vi "DashboardGetvi.vi"(8 "Joystick 2":T1, 9 "Joystick 1":T1) -> ()   [LabVIEW 2018]
uses:
  <vilib>/Rock Robotics/WPI/Joystick/WPI_JoystickDevRef.ctl
  <vilib>/Rock Robotics/WPI/Joystick/WPI_JoystickDeviceEnum.ctl
  <vilib>/Rock Robotics/Network Tables/NT Read Boolean.vi
  <vilib>/Rock Robotics/Network Tables/NT Read Number.vi
  Inputs_DriverStation.vi
  RobotStates.vi
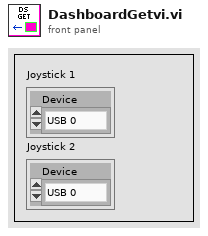
[diagram p1: front panel]
types:
  T1 = typedef "WPI_JoystickDevRef.ctl" = cluster{"Device":T2}
  T2 = typedef "WPI_JoystickDeviceEnum.ctl" = enum16{"USB 0", "USB 1", "USB 2", "USB 3", "USB 4", "USB 5"}
  T3 = cluster{bool, bool, bool, bool, bool, bool, bool, bool, bool, bool, bool, bool, bool, bool}
  T4 = cluster{"Boolean":bool, "Boolean":bool, "Boolean":bool, "Boolean":bool, "Boolean":bool, "Boolean":bool, "Boolean":bool, "Boolean":bool, "Boolean":bool, "Boolean":bool, "Boolean":bool, "Boolean":bool, "Boolean":bool, "Boolean":bool}
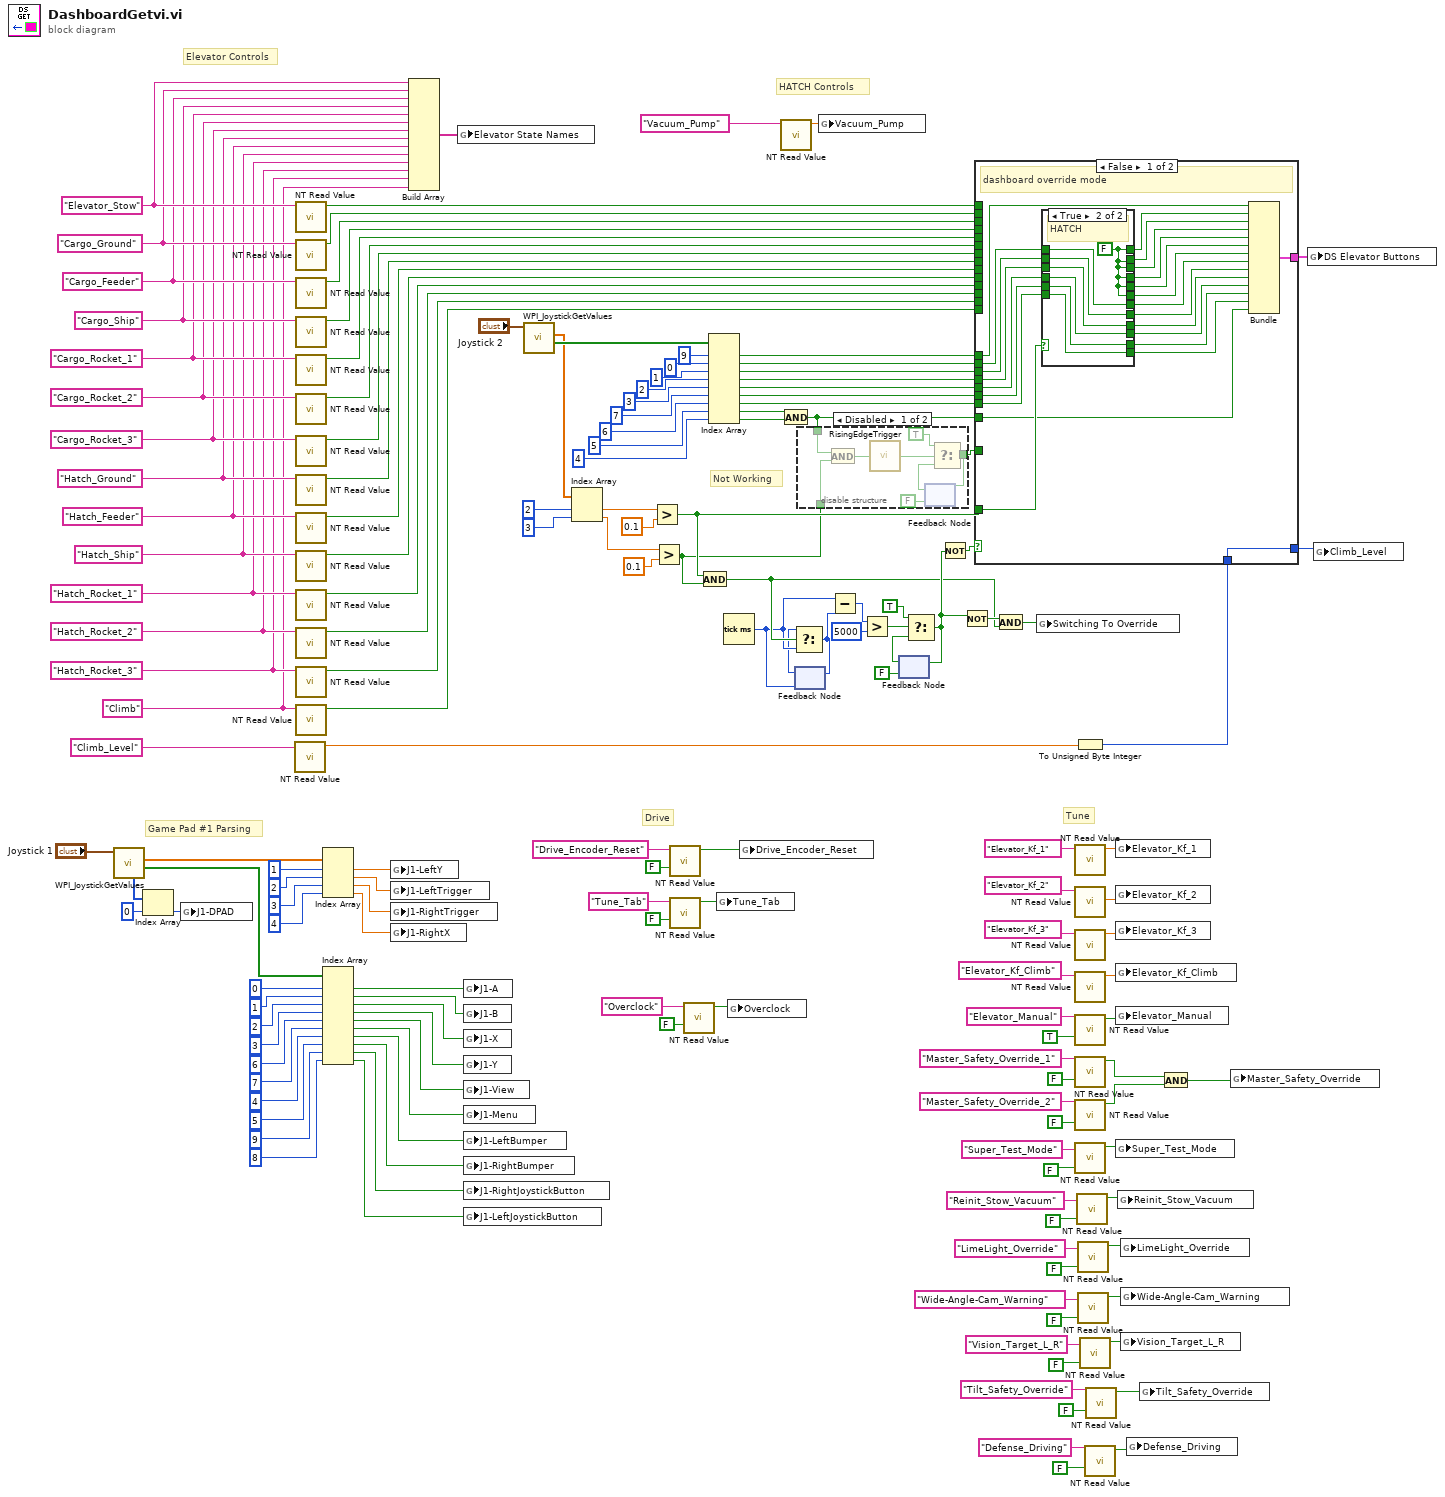
[diagram p0: block diagram]
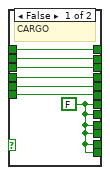
[diagram p3: hidden frame]
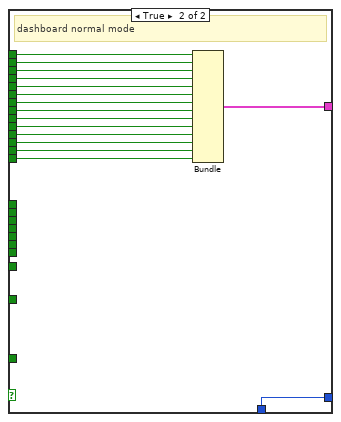
[diagram p4: hidden frame]
diagram:
  w92 = "Climb" ("refnum name")
  w100 = "Hatch_Rocket_3" ("refnum name")
  w101 = "Hatch_Rocket_2" ("refnum name")
  w102 = "Hatch_Rocket_1" ("refnum name")
  w103 = "Hatch_Ship" ("refnum name")
  w104 = "Hatch_Feeder" ("refnum name")
  w105 = "Hatch_Ground" ("refnum name")
  w149 = "Cargo_Rocket_3" ("refnum name")
  w150 = "Cargo_Rocket_2" ("refnum name")
  w151 = "Cargo_Rocket_1" ("refnum name")
  w152 = "Cargo_Ship" ("refnum name")
  w158 = "Cargo_Feeder" ("refnum name")
  w159 = "Cargo_Ground" ("refnum name")
  w160 = "Elevator_Stow" ("refnum name")
  # "Not Working"
  # "Tune"
  # "Drive"
  # "HATCH Controls"
  # "Game Pad #1 Parsing"
  # "Elevator Controls"
  n1 = call <vilib>:"WPI_JoystickGetValues.vi"("JoystickDevRef"="Joystick 1") -> ("Buttons"=w140:bool[], "Axes"=w139:dbl[], "POVs"=w136:i16[])  [unwired: 6 in, 2 out]
  n2 = Index Array(array=w136, index=0) -> (element=w133:i16)
  n3 = global write "Inputs_DriverStation.vi" "J1-DPAD"(w133) -> ()
  n4 = call-poly <vilib>:"NT Read Value.vi"("Name"="Climb_Level" ("refnum name")) -> ("Numeric"=w9:dbl)  [unwired: 9 in, 1 out]
  n5 = call-poly <vilib>:"NT Read Value.vi"("Name"=w160) -> ("Boolean"=w163:bool)  [unwired: 9 in, 1 out]
  n6 = call-poly <vilib>:"NT Read Value.vi"("Name"=w159) -> ("Boolean"=w162:bool)  [unwired: 9 in, 1 out]
  n7 = call-poly <vilib>:"NT Read Value.vi"("Name"=w158) -> ("Boolean"=w161:bool)  [unwired: 9 in, 1 out]
  n8 = call-poly <vilib>:"NT Read Value.vi"("Name"=w152) -> ("Boolean"=w156:bool)  [unwired: 9 in, 1 out]
  n9 = call-poly <vilib>:"NT Read Value.vi"("Name"=w151) -> ("Boolean"=w155:bool)  [unwired: 9 in, 1 out]
  n10 = call-poly <vilib>:"NT Read Value.vi"("Name"=w150) -> ("Boolean"=w154:bool)  [unwired: 9 in, 1 out]
  n11 = call-poly <vilib>:"NT Read Value.vi"("Name"=w149) -> ("Boolean"=w153:bool)  [unwired: 9 in, 1 out]
  n12 = call-poly <vilib>:"NT Read Value.vi"("Name"=w105) -> ("Boolean"=w112:bool)  [unwired: 9 in, 1 out]
  n13 = call-poly <vilib>:"NT Read Value.vi"("Name"=w104) -> ("Boolean"=w111:bool)  [unwired: 9 in, 1 out]
  n14 = call-poly <vilib>:"NT Read Value.vi"("Name"=w103) -> ("Boolean"=w110:bool)  [unwired: 9 in, 1 out]
  n15 = call-poly <vilib>:"NT Read Value.vi"("Name"=w102) -> ("Boolean"=w109:bool)  [unwired: 9 in, 1 out]
  n16 = call-poly <vilib>:"NT Read Value.vi"("Name"=w101) -> ("Boolean"=w108:bool)  [unwired: 9 in, 1 out]
  n17 = call-poly <vilib>:"NT Read Value.vi"("Name"=w100) -> ("Boolean"=w107:bool)  [unwired: 9 in, 1 out]
  n18 = call-poly <vilib>:"NT Read Value.vi"("Name"=w92) -> ("Boolean"=w91:bool)  [unwired: 9 in, 1 out]
  n19 = Index Array(array=w139, index #1=1 ("index"), index #2=2 ("index"), index #3=3 ("index"), index #4=4 ("index")) -> (element #1=w126:dbl, element #2=w127:dbl, element #3=w128:dbl, element #4=w125:dbl)
  n20 = Index Array(array=w140, index #1=0 ("index"), index #2=1 ("index"), index #3=2 ("index"), index #4=3 ("index"), index #5=6 ("index"), index #6=7 ("index"), index #7=4 ("index"), index #8=5 ("index"), index #9=9 ("index"), index #10=8 ("index")) -> (element #1=w132:bool, element #2=w131:bool, element #3=w130:bool, element #4=w129:bool, element #5=w89:bool, element #6=w85:bool, element #7=w82:bool, element #8=w81:bool, element #9=w79:bool, element #10=w74:bool)
  n21 = global write "Inputs_DriverStation.vi" "J1-LeftY"(w126) -> ()
  n22 = global write "Inputs_DriverStation.vi" "J1-LeftTrigger"(w127) -> ()
  n23 = global write "Inputs_DriverStation.vi" "J1-RightTrigger"(w128) -> ()
  n24 = global write "Inputs_DriverStation.vi" "J1-RightX"(w125) -> ()
  n25 = Build Array(w160, w159, w158, w152, w151, w150, w149, w105, w104, w103, w102, w101, w100, w92) -> (w157:string[])
  n26 = global write "RobotStates.vi" "Elevator State Names"(w157) -> ()
  n27 = global write "Inputs_DriverStation.vi" "J1-A"(w132) -> ()
  n28 = global write "Inputs_DriverStation.vi" "J1-B"(w131) -> ()
  n29 = global write "Inputs_DriverStation.vi" "J1-X"(w130) -> ()
  n30 = global write "Inputs_DriverStation.vi" "J1-Y"(w129) -> ()
  n31 = global write "Inputs_DriverStation.vi" "J1-View"(w89) -> ()
  n32 = global write "Inputs_DriverStation.vi" "J1-Menu"(w85) -> ()
  n33 = global write "Inputs_DriverStation.vi" "J1-LeftBumper"(w82) -> ()
  n34 = global write "Inputs_DriverStation.vi" "J1-RightBumper"(w81) -> ()
  n35 = global write "Inputs_DriverStation.vi" "J1-RightJoystickButton"(w79) -> ()
  n36 = global write "Inputs_DriverStation.vi" "J1-LeftJoystickButton"(w74) -> ()
  n37 = call <vilib>:"WPI_JoystickGetValues.vi"("JoystickDevRef"="Joystick 2") -> ("Buttons"=w69:bool[], "Axes"=w53:dbl[])  [unwired: 6 in, 3 out]
  n38 = Index Array(array=w53, index #1=2 ("index"), index #2=3 ("index")) -> (element #1=w52:dbl, element #2=w48:dbl)
  n39 = Greater?(x=w52, y=0.1) -> (0:w47:bool)
  n40 = Greater?(x=w48, y=0.1) -> (0:w35:bool)
  n41 = call-poly <vilib>:"NT Read Value.vi"("Default Value"=FALSE, "Name"="Drive_Encoder_Reset" ("refnum name")) -> ("Boolean"=w113:bool)  [unwired: 8 in, 1 out]
  n42 = call-poly <vilib>:"NT Read Value.vi"("Default Value"=FALSE, "Name"="Tune_Tab" ("refnum name")) -> ("Boolean"=w76:bool)  [unwired: 8 in, 1 out]
  n43 = call-poly <vilib>:"NT Read Value.vi"("Default Value"=FALSE, "Name"="Overclock" ("refnum name")) -> ("Boolean"=w23:bool)  [unwired: 8 in, 1 out]
  n44 = And(x=w47, y=w35) -> (x .and. y?=w29:bool)
  n45 = Index Array(array=w69, index #1=9 ("index"), index #2=0 ("index"), index #3=1 ("index"), index #4=2 ("index"), index #5=3 ("index"), index #6=7 ("index"), index #7=6 ("index"), index #8=5 ("index"), index #9=4 ("index")) -> (element #1=w67:bool, element #2=w65:bool, element #3=w63:bool, element #4=w61:bool, element #5=w59:bool, element #6=w57:bool, element #7=w55:bool, element #8=w38:bool, element #9=w37:bool)
  n46 = global write "Inputs_DriverStation.vi" "Tune_Tab"(w76) -> ()
  n47 = Tick Count (ms)() -> (millisecond timer value=w27:u32)
  n48 = global write "Inputs_DriverStation.vi" "Overclock"(w23) -> ()
  n49 = global write "Inputs_DriverStation.vi" "Drive_Encoder_Reset"(w113) -> ()
  n50 = call-poly <vilib>:"NT Read Value.vi"("Name"="Vacuum_Pump" ("refnum name")) -> ("Numeric"=w116:dbl)  [unwired: 9 in, 1 out]
  n51 = And(x=w38, y=w37) -> (x .and. y?=w36:bool)
  n52 = feedback #1(w27) -> (w26:u32)
  n53 = Select(t=w26, s=w29, f=w27) -> (s? t:f=w33:u32)
  n54 = feedback-in #1(w33) -> ()
  n55 = disable-structure shown="Disabled" {
    disable-tunnel: w36 -> [w171 _]
    disable-tunnel: w35 -> [w170 _]
    disable-tunnel: [w164 _] -> w34
    frame Disabled {
      n56 = And(x=w171, y=w170) -> (x .and. y?=w169:bool)
      n57 = call "RisingEdgeTrigger.vi"("Raw Signal"=w169) -> ("Trigger"=w165:bool)
      n58 = feedback #2(FALSE) -> (w167:bool)
      n59 = Select(t=TRUE, s=w165, f=w167) -> (s? t:f=w164:bool)
      n60 = feedback-in #2(w164) -> ()
    }
    frame Enabled {
    }
  }
  n61 = global write "Inputs_DriverStation.vi" "Vacuum_Pump"(w116) -> ()
  n62 = Subtract(x=w27, y=w33) -> (x-y=w32:u32)
  n63 = Greater?(x=w32, y=u32 5000) -> (0:w45:bool)
  n64 = feedback #3(FALSE) -> (w43:bool)
  n65 = Select(t=TRUE, s=w45, f=w43) -> (s? t:f=w30:bool)
  n66 = feedback-in #3(w30) -> ()
  n67 = Not(x=w30) -> (.not. x?=w41:bool)
  n68 = Not(x=w30) -> (.not. x?=w31:bool)
  n69 = And(x=w31, y=w29) -> (x .and. y?=w28:bool)
  n70 = global write "Inputs_DriverStation.vi" "Switching To Override"(w28) -> ()
  n71 = To Unsigned Byte Integer(number=w9) -> (unsigned 8bit integer=w8:u8)
  n72 = case shown="False" w41 {
    tunnel: w163 -> [_ w224]
    tunnel: w162 -> [_ w223]
    tunnel: w161 -> [_ w222]
    tunnel: w156 -> [_ w221]
    tunnel: w155 -> [_ w220]
    tunnel: w154 -> [_ w219]
    tunnel: w153 -> [_ w218]
    tunnel: w112 -> [_ w217]
    tunnel: w111 -> [_ w216]
    tunnel: w110 -> [_ w215]
    tunnel: w109 -> [_ w214]
    tunnel: w108 -> [_ w213]
    tunnel: w107 -> [_ w212]
    tunnel: [w173 w211] -> w106
    tunnel: w91 -> [_ w210]
    tunnel: w67 -> [w194 _]
    tunnel: w65 -> [w193 _]
    tunnel: w63 -> [w191 _]
    tunnel: w61 -> [w189 _]
    tunnel: w59 -> [w188 _]
    tunnel: w57 -> [w187 _]
    tunnel: w55 -> [w186 _]
    tunnel: w47 -> [w185 _]
    tunnel: w36 -> [w184 _]
    tunnel: [w172 w209] -> w7
    tunnel: w34 -> [_ _]
    tunnel: w8 -> [w172 w209]
    frame False {
      # "dashboard override mode"
      n73 = case shown="True" w185 {
        tunnel: w193 -> [w201 w207]
        tunnel: [w201 w208] -> w192
        tunnel: w191 -> [w200 w206]
        tunnel: [w200 w208] -> w190
        tunnel: w189 -> [w199 w205]
        tunnel: [w199 w208] -> w183
        tunnel: w188 -> [w198 w204]
        tunnel: [w198 w208] -> w182
        tunnel: w187 -> [w197 w203]
        tunnel: [w197 w208] -> w181
        tunnel: w186 -> [w196 w202]
        tunnel: [w196 w208] -> w180
        tunnel: [w195 w207] -> w179
        tunnel: [w195 w206] -> w178
        tunnel: [w195 w205] -> w177
        tunnel: [w195 w204] -> w176
        tunnel: [w195 w203] -> w175
        tunnel: [w195 w202] -> w174
        frame False {
          w195 = FALSE
          # "CARGO"
        }
        frame True {
          w208 = FALSE
          # "HATCH"
        }
      }
      n74 = Bundle(w194, w192, w190, w183, w182, w181, w180, w179, w178, w177, w176, w175, w174, w184) -> (w173:T3)  [unwired: 1 in]
    }
    frame True {
      # "dashboard normal mode"
      n75 = Bundle("Boolean"=w224, "Boolean"=w223, "Boolean"=w222, "Boolean"=w221, "Boolean"=w220, "Boolean"=w219, "Boolean"=w218, "Boolean"=w217, "Boolean"=w216, "Boolean"=w215, "Boolean"=w214, "Boolean"=w213, "Boolean"=w212, "Boolean"=w210) -> (w211:T4)  [unwired: 1 in]
    }
  }
  n76 = call-poly <vilib>:"NT Read Value.vi"("Name"="Elevator_Kf_1" ("refnum name")) -> ("Numeric"=w147:dbl)  [unwired: 9 in, 1 out]
  n77 = call-poly <vilib>:"NT Read Value.vi"("Name"="Elevator_Kf_2" ("refnum name")) -> ("Numeric"=w120:dbl)  [unwired: 9 in, 1 out]
  n78 = call-poly <vilib>:"NT Read Value.vi"("Name"="Elevator_Kf_3" ("refnum name")) -> ("Numeric"=w118:dbl)  [unwired: 9 in, 1 out]
  n79 = call-poly <vilib>:"NT Read Value.vi"("Name"="Elevator_Kf_Climb" ("refnum name")) -> ("Numeric"=w87:dbl)  [unwired: 9 in, 1 out]
  n80 = call-poly <vilib>:"NT Read Value.vi"("Default Value"=TRUE, "Name"="Elevator_Manual" ("refnum name")) -> ("Boolean"=w123:bool)  [unwired: 8 in, 1 out]
  n81 = call-poly <vilib>:"NT Read Value.vi"("Default Value"=FALSE, "Name"="Master_Safety_Override_1" ("refnum name")) -> ("Boolean"=w95:bool)  [unwired: 8 in, 1 out]
  n82 = call-poly <vilib>:"NT Read Value.vi"("Default Value"=FALSE, "Name"="Master_Safety_Override_2" ("refnum name")) -> ("Boolean"=w94:bool)  [unwired: 8 in, 1 out]
  n83 = call-poly <vilib>:"NT Read Value.vi"("Default Value"=FALSE, "Name"="Super_Test_Mode" ("refnum name")) -> ("Boolean"=w72:bool)  [unwired: 8 in, 1 out]
  n84 = call-poly <vilib>:"NT Read Value.vi"("Default Value"=FALSE, "Name"="Reinit_Stow_Vacuum" ("refnum name")) -> ("Boolean"=w21:bool)  [unwired: 8 in, 1 out]
  n85 = call-poly <vilib>:"NT Read Value.vi"("Default Value"=FALSE, "Name"="LimeLight_Override" ("refnum name")) -> ("Boolean"=w18:bool)  [unwired: 8 in, 1 out]
  n86 = call-poly <vilib>:"NT Read Value.vi"("Default Value"=FALSE, "Name"="Wide-Angle-Cam_Warning" ("refnum name")) -> ("Boolean"=w14:bool)  [unwired: 8 in, 1 out]
  n87 = call-poly <vilib>:"NT Read Value.vi"("Default Value"=FALSE, "Name"="Vision_Target_L_R" ("refnum name")) -> ("Boolean"=w11:bool)  [unwired: 8 in, 1 out]
  n88 = call-poly <vilib>:"NT Read Value.vi"("Default Value"=FALSE, "Name"="Defense_Driving" ("refnum name")) -> ("Boolean"=w2:bool)  [unwired: 8 in, 1 out]
  n89 = call-poly <vilib>:"NT Read Value.vi"("Default Value"=FALSE, "Name"="Tilt_Safety_Override" ("refnum name")) -> ("Boolean"=w4:bool)  [unwired: 8 in, 1 out]
  n90 = global write "Inputs_DriverStation.vi" "Elevator_Kf_1"(w147) -> ()
  n91 = global write "Inputs_DriverStation.vi" "Elevator_Kf_2"(w120) -> ()
  n92 = global write "Inputs_DriverStation.vi" "Elevator_Kf_3"(w118) -> ()
  n93 = global write "Inputs_DriverStation.vi" "Elevator_Kf_Climb"(w87) -> ()
  n94 = global write "Inputs_DriverStation.vi" "Elevator_Manual"(w123) -> ()
  n95 = global write "Inputs_DriverStation.vi" "Super_Test_Mode"(w72) -> ()
  n96 = global write "Inputs_DriverStation.vi" "Reinit_Stow_Vacuum"(w21) -> ()
  n97 = global write "Inputs_DriverStation.vi" "LimeLight_Override"(w18) -> ()
  n98 = global write "Inputs_DriverStation.vi" "Wide-Angle-Cam_Warning"(w14) -> ()
  n99 = global write "Inputs_DriverStation.vi" "Vision_Target_L_R"(w11) -> ()
  n100 = global write "Inputs_DriverStation.vi" "Defense_Driving"(w2) -> ()
  n101 = global write "Inputs_DriverStation.vi" "Tilt_Safety_Override"(w4) -> ()
  n102 = And(x=w95, y=w94) -> (x .and. y?=w93:bool)
  n103 = global write "Inputs_DriverStation.vi" "Master_Safety_Override"(w93) -> ()
  n104 = global write "Inputs_DriverStation.vi" "DS Elevator Buttons"(w106) -> ()
  n105 = global write "Inputs_DriverStation.vi" "Climb_Level"(w7) -> ()
